vi "RSNRPZ Measurement Mode.vi"(8 "error in (no error)":errorcluster, 9 "Measurement Mode (ContAv)":i32(ring) items=["ContAv"=0, "Buffered ContAv"=1, "Timeslot"=2, "Burst"=3, "Scope"=4, "CCDF"=6, "PDF"=7], 10 "Channel (1)":i32=1, 11 "VISA session":refnum<visa-resource-name> caption="VISA resource name") -> (0 "error out":errorcluster, 3 "dup VISA session":refnum<visa-resource-name> caption="VISA resource name")   [LabVIEW 2019]
doc: "This VI sets the sensor to one of the measurement modes.\n\nRemote-control command(s):\nSENSe[1..4]:FUNCtion\nSENSe[1..4]:BUFFer:STATe ON | OFF"
uses:
  rsnrpz_32.dll
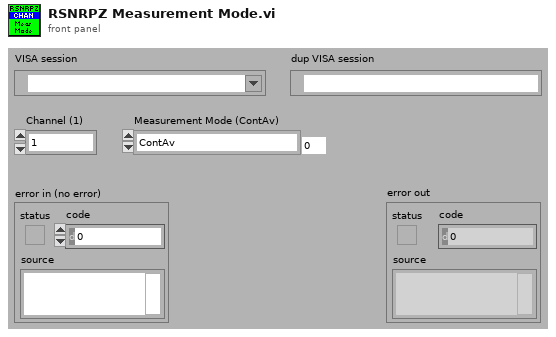
[diagram p1: front panel]
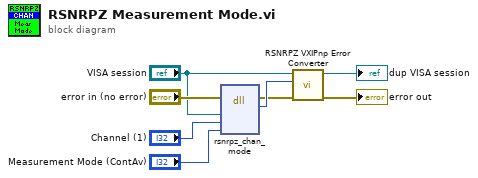
[diagram p0: block diagram]
diagram:
  n1 = dll-call lib="C:/Users/LABadmin/Documents/Jarvis/user_lib/rsnrpz/rsnrpz_32.dll" fn="rsnrpz_chan_mode"(error in="error in (no error)", "VISA Session"="VISA session", "Channel"="Channel (1)", "Measurement Mode"="Measurement Mode (ContAv)") -> (error out=w5:errorcluster, "Status"=w8:i32)  [unwired: 5 in, 1 out]
  n2 = call <instrlib>:"RSNRPZ VXIPnp Error Converter.vi"("error in"=w5, "VXIPnp error code"=w8, "VISA session"="VISA session") -> ("error out"=→"error out":errorcluster, "dup VISA session"=→"dup VISA session":refnum<visa-resource-name>)  [unwired: 7 in]
